vi "AuMT8852B EDR Maximum Input Power Configuration.vi"(5 "Settings":T1={"Low frequency selection"=enum."Use low frequency", "Medium frequency selection"=enum."Use medium frequency", "High frequency selection"=enum."Use high frequency", "Low TX frequency"=2480.0, "Low RX frequency"=2402.0, "Medium TX frequency"=2402.0, "Medium RX frequency"=2441.0, "High TX frequency"=2402.0, "High RX frequency"=2480.0, "Number of bits"=0.1, "2DHx test packet"=enum."OFF", "3DHx test packet"=enum."OFF", "Hop selection"=enum."Test with hopping off and on", "Test TX power"=-70.0, "Overall BER limit"=1, "Packet count"=enum."TX"} {"Test TX power" format="%.1f"; "Number of bits" format="%.2f"}, 7 "Set/Get (Set)":enum16{"Set", "Get"}(ring), 8 "error in (no error)":errorcluster, 10 "Script (3)":i32=3, 11 "VISA session":refnum<visa-resource-name>) -> (0 "error out":errorcluster, 2 "error code":i32, 3 "VISA session out":refnum<visa-resource-name>, 4 "Settings out":T1={"Low frequency selection"=enum."Use low frequency", "Medium frequency selection"=enum."Use medium frequency", "High frequency selection"=enum."Use high frequency", "Low TX frequency"=2480.0, "Low RX frequency"=2402.0, "Medium TX frequency"=2402.0, "Medium RX frequency"=2441.0, "High TX frequency"=2402.0, "High RX frequency"=2480.0, "Number of bits"=0.1, "2DHx test packet"=enum."OFF", "3DHx test packet"=enum."OFF", "Hop selection"=enum."Test with hopping off and on", "Test TX power"=-70.0, "Overall BER limit"=1, "Packet count"=enum."TX"} {"Test TX power" format="%.1f"; "Number of bits" format="%.2f"})   [LabVIEW 2017]
doc: "Anritsu MT8852B Bluetooth Tester\n\nConfigures the instrument for the EDR Maximum Input Power test.\n\nINPUTS\nSet/Get - whether the values are being sent to or retrieved from the instrument.\nScript - which of the stored scripts (1-10) will be queried or configured. Scripts 1 and 2 are read-only.\nSettings - parameters of the test to be written.\n\nOUTPUTS\nSettings out - current parameters of the test."
uses:
  <instrlib>/aumt8852B/General/Utilities/MT8850 Test Parameters.ctl
  <instrlib>/aumt8852B/General/Utilities/MT8850 Frequency Units.ctl
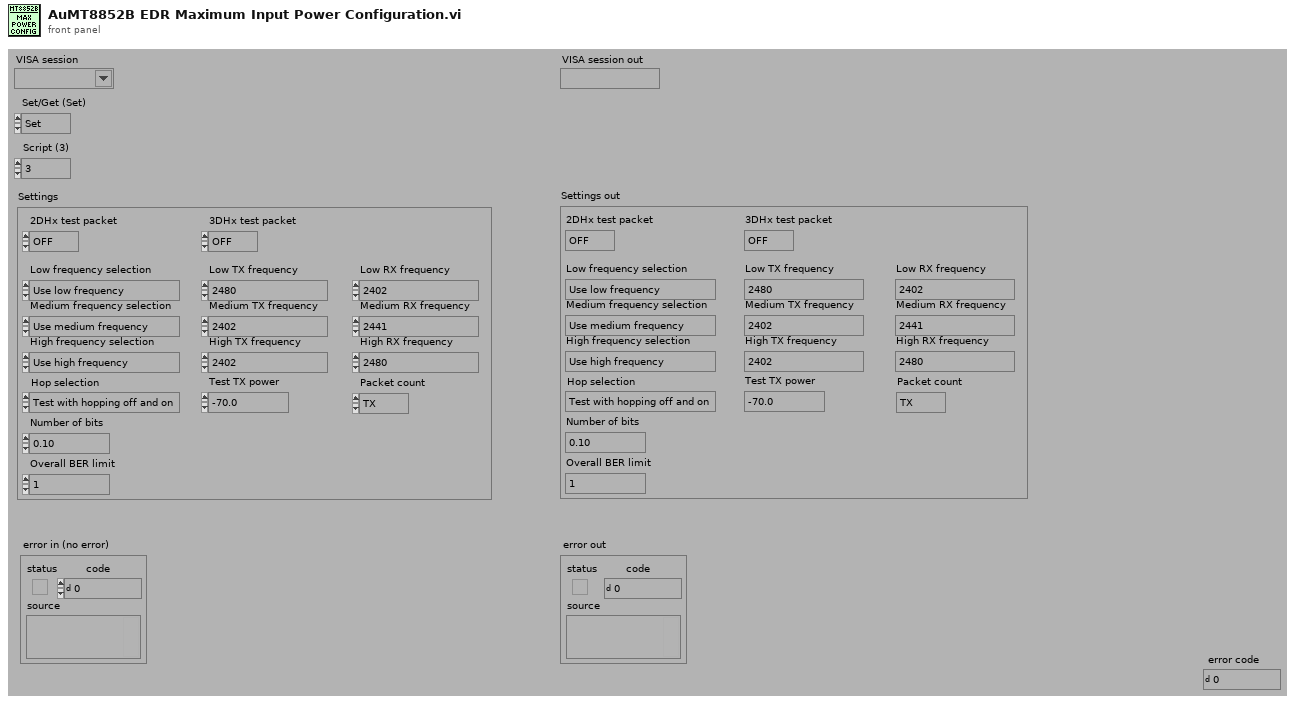
[diagram p1: front panel]
types:
  T1 = cluster{"Low frequency selection":enum16{"Don't use low frequency", "Use low frequency"}, "Medium frequency selection":enum16{"Don't use medium frequency", "Use medium frequency"}, "High frequency selection":enum16{"Don't use high frequency", "Use high frequency"}, "Low TX frequency":dbl, "Low RX frequency":dbl, "Medium TX frequency":dbl, "Medium RX frequency":dbl, "High TX frequency":dbl, "High RX frequency":dbl, "Number of bits":dbl, "2DHx test packet":enum16{"OFF", "Longest", "2-DH1", "2-DH3", "2-DH5"}, "3DHx test packet":enum16{"OFF", "Longest", "3-DH1", "3-DH3", "3-DH5"}, "Hop selection":enum16{"Test with hopping on", "Test with hopping off", "Test with hopping off and on"}, "Test TX power":dbl, "Overall BER limit":i16, "Packet count":enum16{"TX", "RX"}}
  T2 = typedef "MT8850 Test Parameters.ctl" = enum16{"Use low frequency", "Use medium frequency", "Use high frequency", "Low TX frequency", "Low RX frquency", "Medium TX frequency", "Medium RX frequency", "High TX frequency", "High RX frequency", "Number of packets", "Average high limit", "Average low limit", "Peak power limit", "Max power step limit", "Min power step limit", "f1 average minimum", "f1 average maximum", "f2 maximum", "f1/f2 average maximum", "Hop selection", "Use DH1 packets", "Use DH3 packets", "Use DH5 packets", "1 slot packet drift limit", "3 slot packet drift limit", "5 slot packet drift limit", "Drift rate limit", "TX power level", "Frequency offset", "Symbol timing", "Modulation index", "BER limit", "FER limit", "Use averaging high limit", "Use averaging low limit", "Use peak power limit", "Packet type", "Test control", "Use max power step limit", "Use min power step limit", "Number of cycles", "Use f1 average maximum", "Use f1 average minimum", "Use f2 maximum", "Use f1/f2 average maximum", "Hop mode", "Maximum negative limit", "Maximum positive limit", "Use maximum negative limit", "Use maximum positive limit", "Use 1 slot packet drift limit", "Use 3 slot packet drift limit", "Use 5 slot packet drift limit", "Use drift rate limit", "Use BER limit", "Use FER limit", "Use dirty parameter table", "Use null packet drift limit", "Null packet drift limit", "Minimum power", "Power delay", "Packet count", "Payload toggle", "Output power level", "2DHX packet type", "3DHX packet type", "Number of blocks", "TX and RX low frequency", "TX and RX medium frequency", "TX and RX high frequency", "TX frequency", "RX frequency", "Threshold bit count", "Total test bit count", "Number of bits", "PDPSK to PGFSK lower limit", "PDPSK to PGFSK upper limit", "Initial frequency error upper limit", "Initial frequency error lower limit", "Frequency error upper limit", "Frequency error lower limit", "Block frequency error upper limit", "Block frequency error lower limit", "2Mbs RMS DEVM limit", "3Mbs RMS DEVM limit", "2Mbs Peak DEVM limit", "3Mbs Peak DEVM limit", "2Mbs 99% packets DEVM limit", "3Mbs 99% packets DEVM limit", "Percentage of no error packets limit", "Threshold error limit", "Total test error limit"}
  T3 = enum16{"Output power", "Power control", "Modulation characteristics", "Initial carrier", "Carrier drift", "Single slot sensitivity", "Multiple slot sensitivity", "Maximum input power", "EDR Relative transmit power", "EDR Carrier frequency and stability", "EDR Differential phase encoding", "EDR Sensitivity", "EDR BER floor sensitivity", "EDR Maximum input power"}
  T4 = typedef "MT8850 Frequency Units.ctl" = enum16{"Channel", "Hz", "kHz", "MHz", "GHz"}
  T5 = enum16{"Simulate", "Range check", "Cache", "Query instrument status"}
  T6 = enum16{"Test with hopping on", "Test with hopping off", "Test with hopping off and on"}
  T7 = enum16{"OFF", "Longest", "3-DH1", "3-DH3", "3-DH5"}
  T8 = enum16{"OFF", "Longest", "2-DH1", "2-DH3", "2-DH5"}
  T9 = enum16{"Don't use high frequency", "Use high frequency"}
  T10 = enum16{"Don't use medium frequency", "Use medium frequency"}
  T11 = enum16{"Don't use low frequency", "Use low frequency"}
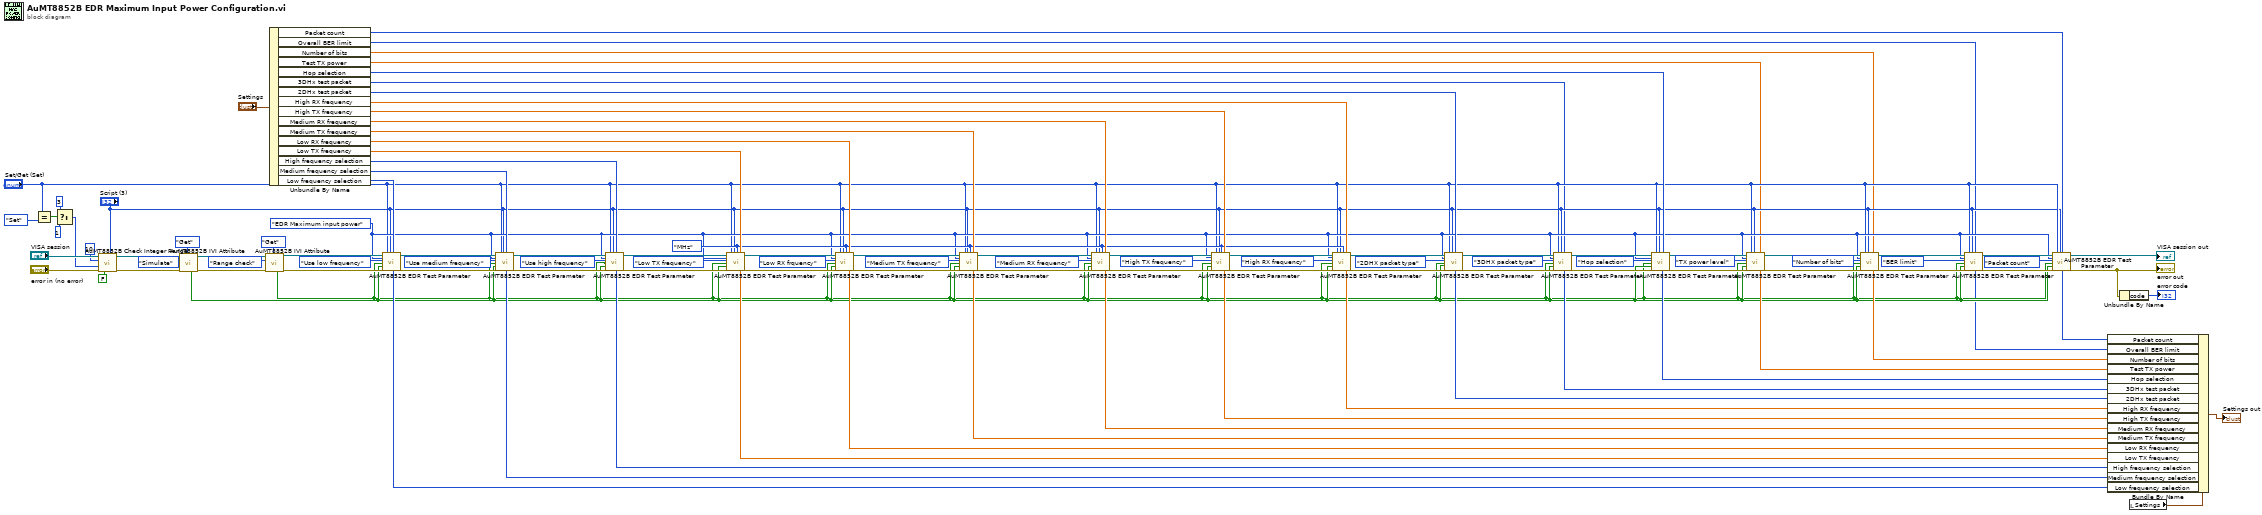
[diagram p0: block diagram]
diagram:
  w12 = T3."EDR Maximum input power" ("Test (Output power)")
  w37 = MT8850_Frequency_Units."MHz" ("Frequency units (MHz)")
  n1 = Equal?(x="Set/Get (Set)", y=enum16{"Set", "Get"}."Set") -> (x = y?=w106:bool)
  n2 = Select(t=3, s=w106, f=1) -> (s? t:f=w102:i32)
  n3 = call <instrlib>:"AuMT8852B Check Integer Range.vi"("Value (0)"="Script (3)", "Check IVI flag first? (T)"=FALSE, "error in (no error)"="error in (no error)", "Lower limit (-1)"=w102, "Upper limit (1)"=10, "VISA session"="VISA session") -> ("error out"=w100:errorcluster, "VISA session out"=w101:refnum<visa-resource-name>)  [unwired: 4 in]
  n4 = call <instrlib>:"AuMT8852B IVI Attribute.vi"("Set/Get (Set)"=enum16{"Set", "Get"}."Get", "error in (no error)"=w100, "Flag (Simulate)"=T5."Simulate", "VISA session"=w101) -> ("error out"=w74:errorcluster, "VISA session out"=w75:refnum<visa-resource-name>, "Value out"=w7:bool)  [unwired: 5 in]
  n5 = call <instrlib>:"AuMT8852B IVI Attribute.vi"("Set/Get (Set)"=enum16{"Set", "Get"}."Get", "error in (no error)"=w74, "Flag (Simulate)"=T5."Range check", "VISA session"=w75) -> ("error out"=w72:errorcluster, "VISA session out"=w73:refnum<visa-resource-name>, "Value out"=w6:bool)  [unwired: 5 in]
  n6 = Unbundle By Name("Settings") -> ("Packet count"=w8:enum16{"TX", "RX"}, "Overall BER limit"=w4:i16, "Number of bits"=w5:dbl, "Test TX power"=w1:dbl, "Hop selection"=w31:T6, "3DHx test packet"=w2:T7, "2DHx test packet"=w50:T8, "High RX frequency"=w62:dbl, "High TX frequency"=w63:dbl, "Medium RX frequency"=w51:dbl, "Medium TX frequency"=w64:dbl, "Low RX frequency"=w65:dbl, "Low TX frequency"=w66:dbl, "High frequency selection"=w67:T9, "Medium frequency selection"=w68:T10, "Low frequency selection"=w69:T11)
  n7 = call <instrlib>:"AuMT8852B EDR Test Parameter.vi"("VISA session"=w73, "Test (Output power)"=w12, "Parameter (Use low frequency)"=MT8850_Test_Parameters."Use low frequency", "Range check? (F)"=w6, "Simulate? (F)"=w7, "error in (no error)"=w72, "Set/Get (Set)"="Set/Get (Set)", "Script (3)"="Script (3)", "Integer value (0)"=w69) -> ("Integer value out"=w54:i32, "VISA session out"=w43:refnum<visa-resource-name>, "error out"=w42:errorcluster)  [unwired: 7 in, 1 out]
  n8 = call <instrlib>:"AuMT8852B EDR Test Parameter.vi"("VISA session"=w43, "Test (Output power)"=w12, "Parameter (Use low frequency)"=MT8850_Test_Parameters."Use medium frequency", "Range check? (F)"=w6, "Simulate? (F)"=w7, "error in (no error)"=w42, "Set/Get (Set)"="Set/Get (Set)", "Script (3)"="Script (3)", "Integer value (0)"=w68) -> ("Integer value out"=w55:i32, "VISA session out"=w41:refnum<visa-resource-name>, "error out"=w40:errorcluster)  [unwired: 7 in, 1 out]
  n9 = call <instrlib>:"AuMT8852B EDR Test Parameter.vi"("VISA session"=w41, "Test (Output power)"=w12, "Parameter (Use low frequency)"=MT8850_Test_Parameters."Use high frequency", "Range check? (F)"=w6, "Simulate? (F)"=w7, "error in (no error)"=w40, "Set/Get (Set)"="Set/Get (Set)", "Script (3)"="Script (3)", "Integer value (0)"=w67) -> ("Integer value out"=w56:i32, "VISA session out"=w96:refnum<visa-resource-name>, "error out"=w95:errorcluster)  [unwired: 7 in, 1 out]
  n10 = call <instrlib>:"AuMT8852B EDR Test Parameter.vi"("VISA session"=w96, "Test (Output power)"=w12, "Parameter (Use low frequency)"=MT8850_Test_Parameters."Low TX frequency", "Range check? (F)"=w6, "Simulate? (F)"=w7, "error in (no error)"=w95, "Set/Get (Set)"="Set/Get (Set)", "Script (3)"="Script (3)", "Integer value (0)"=w37, "Float value (0)"=w66) -> ("Float value out"=w57:dbl, "VISA session out"=w94:refnum<visa-resource-name>, "error out"=w93:errorcluster)  [unwired: 6 in, 1 out]
  n11 = call <instrlib>:"AuMT8852B EDR Test Parameter.vi"("VISA session"=w94, "Test (Output power)"=w12, "Parameter (Use low frequency)"=MT8850_Test_Parameters."Low RX frquency", "Range check? (F)"=w6, "Simulate? (F)"=w7, "error in (no error)"=w93, "Set/Get (Set)"="Set/Get (Set)", "Script (3)"="Script (3)", "Integer value (0)"=w37, "Float value (0)"=w65) -> ("Float value out"=w58:dbl, "VISA session out"=w92:refnum<visa-resource-name>, "error out"=w91:errorcluster)  [unwired: 6 in, 1 out]
  n12 = call <instrlib>:"AuMT8852B EDR Test Parameter.vi"("VISA session"=w92, "Test (Output power)"=w12, "Parameter (Use low frequency)"=MT8850_Test_Parameters."Medium TX frequency", "Range check? (F)"=w6, "Simulate? (F)"=w7, "error in (no error)"=w91, "Set/Get (Set)"="Set/Get (Set)", "Script (3)"="Script (3)", "Integer value (0)"=w37, "Float value (0)"=w64) -> ("Float value out"=w59:dbl, "VISA session out"=w90:refnum<visa-resource-name>, "error out"=w89:errorcluster)  [unwired: 6 in, 1 out]
  n13 = call <instrlib>:"AuMT8852B EDR Test Parameter.vi"("VISA session"=w90, "Test (Output power)"=w12, "Parameter (Use low frequency)"=MT8850_Test_Parameters."Medium RX frequency", "Range check? (F)"=w6, "Simulate? (F)"=w7, "error in (no error)"=w89, "Set/Get (Set)"="Set/Get (Set)", "Script (3)"="Script (3)", "Integer value (0)"=w37, "Float value (0)"=w51) -> ("Float value out"=w53:dbl, "VISA session out"=w88:refnum<visa-resource-name>, "error out"=w87:errorcluster)  [unwired: 6 in, 1 out]
  n14 = call <instrlib>:"AuMT8852B EDR Test Parameter.vi"("VISA session"=w88, "Test (Output power)"=w12, "Parameter (Use low frequency)"=MT8850_Test_Parameters."High TX frequency", "Range check? (F)"=w6, "Simulate? (F)"=w7, "error in (no error)"=w87, "Set/Get (Set)"="Set/Get (Set)", "Script (3)"="Script (3)", "Integer value (0)"=w37, "Float value (0)"=w63) -> ("Float value out"=w60:dbl, "VISA session out"=w86:refnum<visa-resource-name>, "error out"=w85:errorcluster)  [unwired: 6 in, 1 out]
  n15 = call <instrlib>:"AuMT8852B EDR Test Parameter.vi"("VISA session"=w86, "Test (Output power)"=w12, "Parameter (Use low frequency)"=MT8850_Test_Parameters."High RX frequency", "Range check? (F)"=w6, "Simulate? (F)"=w7, "error in (no error)"=w85, "Set/Get (Set)"="Set/Get (Set)", "Script (3)"="Script (3)", "Integer value (0)"=w37, "Float value (0)"=w62) -> ("Float value out"=w61:dbl, "VISA session out"=w84:refnum<visa-resource-name>, "error out"=w83:errorcluster)  [unwired: 6 in, 1 out]
  n16 = call <instrlib>:"AuMT8852B EDR Test Parameter.vi"("VISA session"=w84, "Test (Output power)"=w12, "Parameter (Use low frequency)"=MT8850_Test_Parameters."2DHX packet type", "Range check? (F)"=w6, "Simulate? (F)"=w7, "error in (no error)"=w83, "Set/Get (Set)"="Set/Get (Set)", "Script (3)"="Script (3)", "Integer value (0)"=w50) -> ("Integer value out"=w52:i32, "VISA session out"=w46:refnum<visa-resource-name>, "error out"=w45:errorcluster)  [unwired: 7 in, 1 out]
  n17 = call <instrlib>:"AuMT8852B EDR Test Parameter.vi"("VISA session"=w46, "Test (Output power)"=w12, "Parameter (Use low frequency)"=MT8850_Test_Parameters."3DHX packet type", "Range check? (F)"=w6, "Simulate? (F)"=w7, "error in (no error)"=w45, "Set/Get (Set)"="Set/Get (Set)", "Script (3)"="Script (3)", "Integer value (0)"=w2) -> ("Integer value out"=w25:i32, "VISA session out"=w34:refnum<visa-resource-name>, "error out"=w35:errorcluster)  [unwired: 7 in, 1 out]
  n18 = call <instrlib>:"AuMT8852B EDR Test Parameter.vi"("VISA session"=w34, "Test (Output power)"=w12, "Parameter (Use low frequency)"=MT8850_Test_Parameters."Hop selection", "Range check? (F)"=w6, "Simulate? (F)"=w7, "error in (no error)"=w35, "Set/Get (Set)"="Set/Get (Set)", "Script (3)"="Script (3)", "Integer value (0)"=w31) -> ("Integer value out"=w24:i32, "VISA session out"=w33:refnum<visa-resource-name>, "error out"=w36:errorcluster)  [unwired: 7 in, 1 out]
  n19 = call <instrlib>:"AuMT8852B EDR Test Parameter.vi"("VISA session"=w33, "Test (Output power)"=w12, "Parameter (Use low frequency)"=MT8850_Test_Parameters."TX power level", "Range check? (F)"=w6, "Simulate? (F)"=w7, "error in (no error)"=w36, "Set/Get (Set)"="Set/Get (Set)", "Script (3)"="Script (3)", "Float value (0)"=w1) -> ("Float value out"=w23:dbl, "VISA session out"=w28:refnum<visa-resource-name>, "error out"=w30:errorcluster)  [unwired: 7 in, 1 out]
  n20 = call <instrlib>:"AuMT8852B EDR Test Parameter.vi"("VISA session"=w28, "Test (Output power)"=w12, "Parameter (Use low frequency)"=MT8850_Test_Parameters."Number of bits", "Range check? (F)"=w6, "Simulate? (F)"=w7, "error in (no error)"=w30, "Set/Get (Set)"="Set/Get (Set)", "Script (3)"="Script (3)", "Float value (0)"=w5) -> ("Float value out"=w21:dbl, "VISA session out"=w27:refnum<visa-resource-name>, "error out"=w29:errorcluster)  [unwired: 7 in, 1 out]
  n21 = call <instrlib>:"AuMT8852B EDR Test Parameter.vi"("VISA session"=w27, "Test (Output power)"=w12, "Parameter (Use low frequency)"=MT8850_Test_Parameters."BER limit", "Range check? (F)"=w6, "Simulate? (F)"=w7, "error in (no error)"=w29, "Set/Get (Set)"="Set/Get (Set)", "Script (3)"="Script (3)", "Integer value (0)"=w4) -> ("Integer value out"=w3:i32, "VISA session out"=w14:refnum<visa-resource-name>, "error out"=w17:errorcluster)  [unwired: 7 in, 1 out]
  n22 = call <instrlib>:"AuMT8852B EDR Test Parameter.vi"("VISA session"=w14, "Test (Output power)"=w12, "Parameter (Use low frequency)"=MT8850_Test_Parameters."Packet count", "Range check? (F)"=w6, "Simulate? (F)"=w7, "error in (no error)"=w17, "Set/Get (Set)"="Set/Get (Set)", "Script (3)"="Script (3)", "Integer value (0)"=w8) -> ("Integer value out"=w13:i32, "VISA session out"=→"VISA session out":refnum<visa-resource-name>, "error out"=w16:errorcluster)  [unwired: 7 in, 1 out]
  "error out" <- w16
  n23 = Unbundle By Name(w16) -> ("code"=→"error code":i32)
  n24 = local read "Settings"() -> (w19:T1)
  n25 = Bundle By Name(cluster=w19, "Packet count"=w13, "Overall BER limit"=w3, "Number of bits"=w21, "Test TX power"=w23, "Hop selection"=w24, "3DHx test packet"=w25, "2DHx test packet"=w52, "High RX frequency"=w61, "High TX frequency"=w60, "Medium RX frequency"=w53, "Medium TX frequency"=w59, "Low RX frequency"=w58, "Low TX frequency"=w57, "High frequency selection"=w56, "Medium frequency selection"=w55, "Low frequency selection"=w54) -> (→"Settings out":T1)
